vi "Frame Configuration Page.vi"(8 "error in (no error)":errorcluster, 11 "Node Ptr":T2 format="%.0x") -> (0 "error out":errorcluster)   [LabVIEW 2016, in "LIN Frame Protection Addon System Explorer.lvlib"]
uses:
  LIN Frame Protection Addon System Explorer.lvlib
  <vilib>/NI Veristand/Custom Device API/Custom Device Item Ref.ctl
  Shared/Types/Protection Type.ctl
  <vilib>/NI Veristand/Custom Device API/Custom Device API.lvlib
  Shared/LIN Frame Protection Addon Shared.lvlib
panel:
  in  "Protection Type":T1
  out "Frame ID":u32 format="%.0x"
  in  "Max Count":dbl=4.0
  out "Frame Rate":dbl
  out "Rolling Counter Channel":string
  out "CRC Channel":string
  in  "SHDocVw.IWebBrowser":refnum<k7>(container)
  in  "Value":dbl
  in  "Monitored Channels":i32(listbox)
  in  "Header":cluster{"Section Name":string}={"Section Name"="Custom Device Item Settings"}
  in  "Description":string
  in  "Name":string
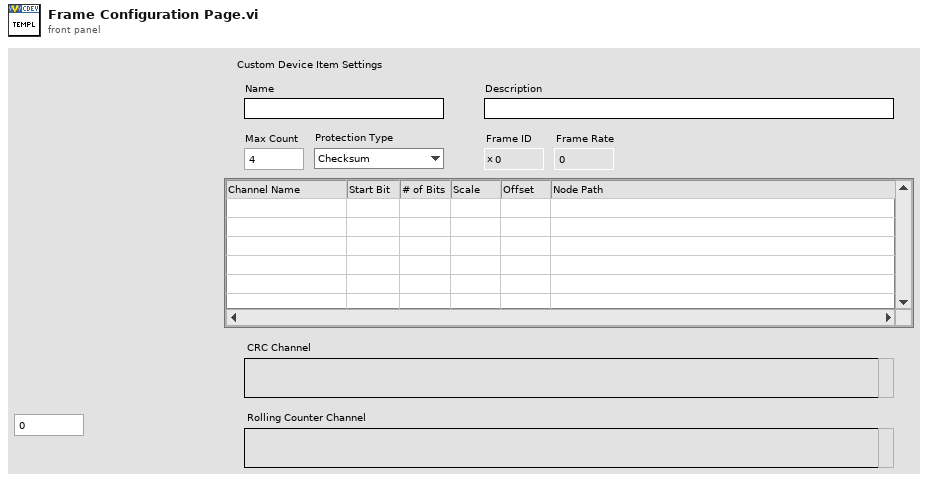
[diagram p1: front panel]
types:
  T1 = typedef "LIN Frame Protection Addon Shared.lvlib/Protection Type.ctl" = enum16{"Checksum", "CRC", "None (Counter Only)"}
  T2 = typedef "Custom Device API.lvlib/Custom Device Item Ref.ctl" = u64
  T3 = typedef "Custom Device API.lvlib/Custom Device Item Info.ctl" = cluster{"Name":string, "Is Channel":bool, "GUID":string, "Is Waveform":bool}
  T4 = typedef "LIN Frame Protection Addon Shared.lvlib/FrameConfiguration.ctl" = cluster{"Input Channels":T5[], "Schedule_SumOfDelays":dbl, "Rolling Counter Count":dbl, "PCL Count":u64, "Max Count":dbl, "Frame ID":u32, "Rolling Counter":T5, "CRC":T5, "Frame Name":string, "Cluster":string, "Database":string, "Protection Type":T1}
  T5 = typedef "LIN Frame Protection Addon Shared.lvlib/InputChannelConfiguration.ctl" = cluster{"Start Bit":i32, "Name":string, "Node Path":string, "Number of bits":i32, "Scale":dbl, "Offset":dbl, "Data Type":u32}
  T6 = typedef "Custom Device API.lvlib/Custom Device Commands.ctl" = enum16{"Default", "Item renamed", "Shutdown", "Dynamic button pressed"}
  T7 = typedef "LVPoint32TypeDef.ctl" = cluster{"Horizontal":i32, "Vertical":i32}
  T8 = typedef "LVRowAndColumnTypeDef.ctl" = cluster{"Row":i32, "Column":i32}
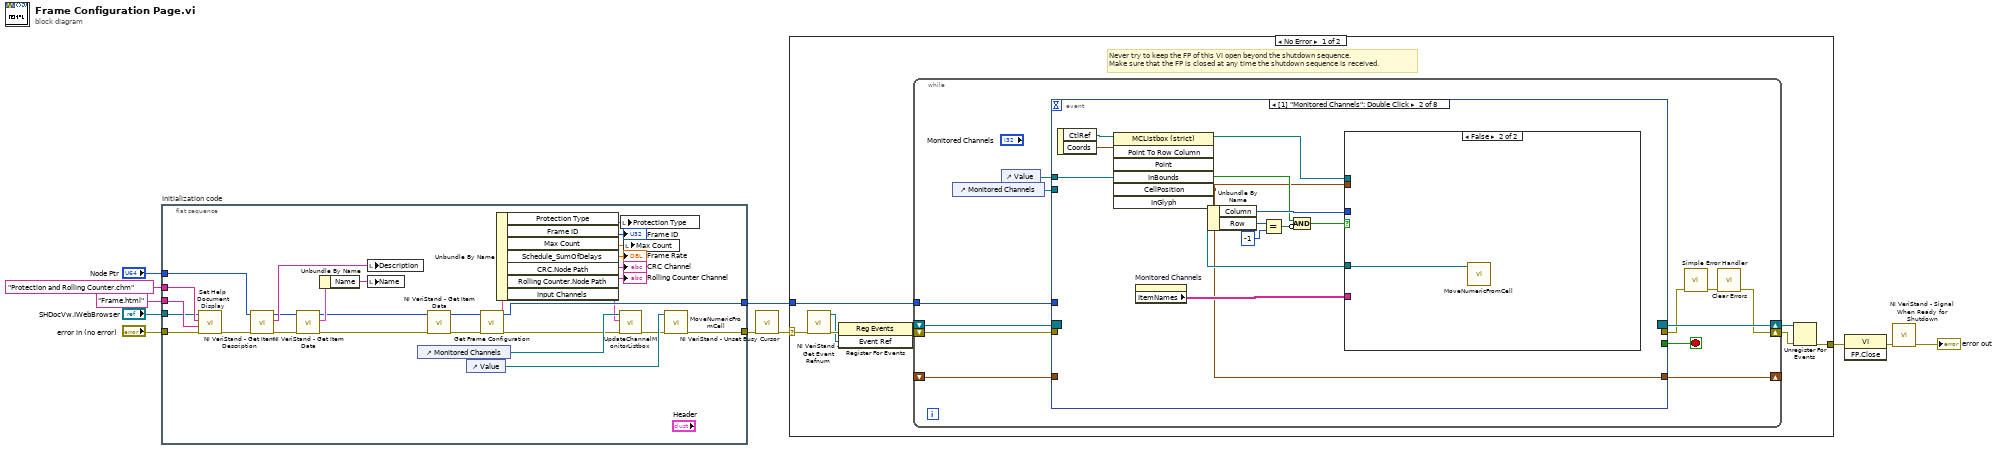
[diagram p0: block diagram]
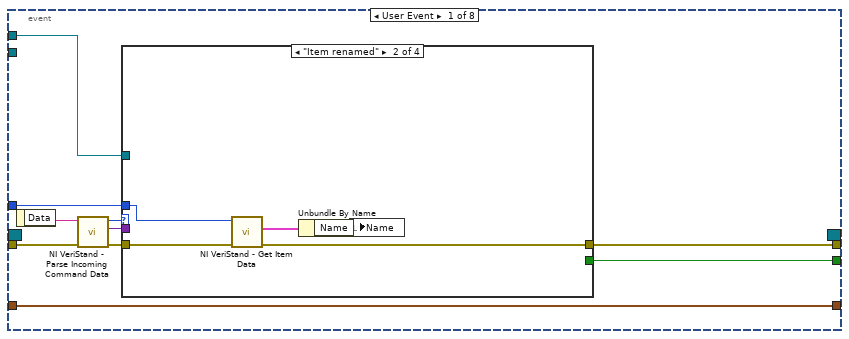
[diagram p2: hidden frame]
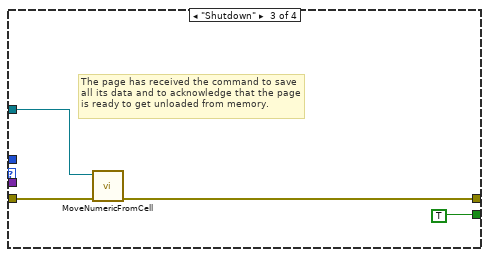
[diagram p4: hidden frame]
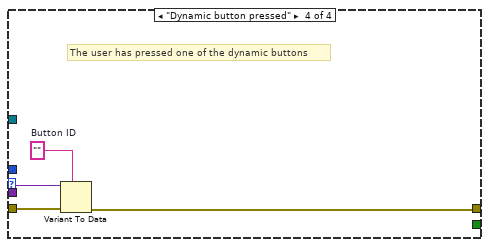
[diagram p5: hidden frame]
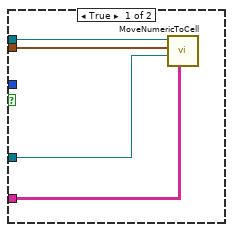
[diagram p6: hidden frame]
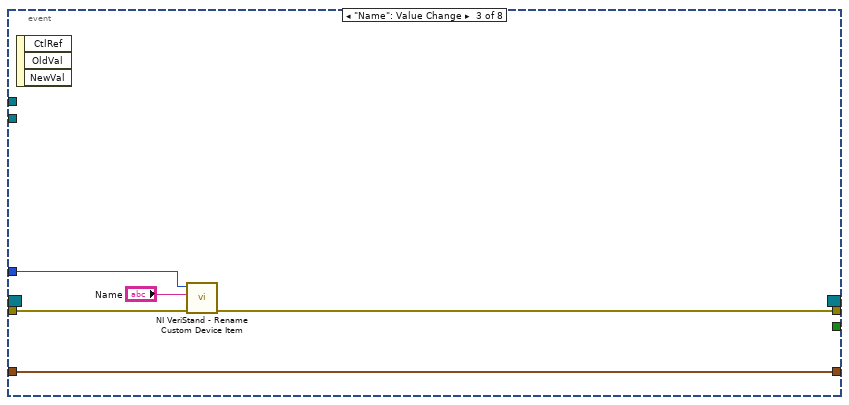
[diagram p7: hidden frame]
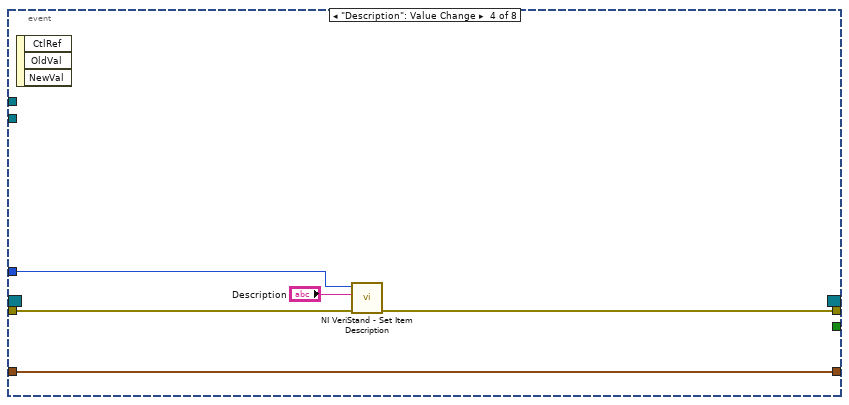
[diagram p8: hidden frame]
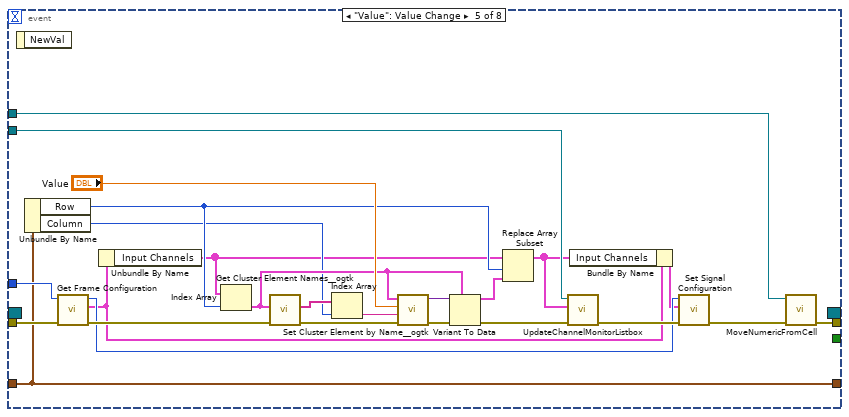
[diagram p9: hidden frame]
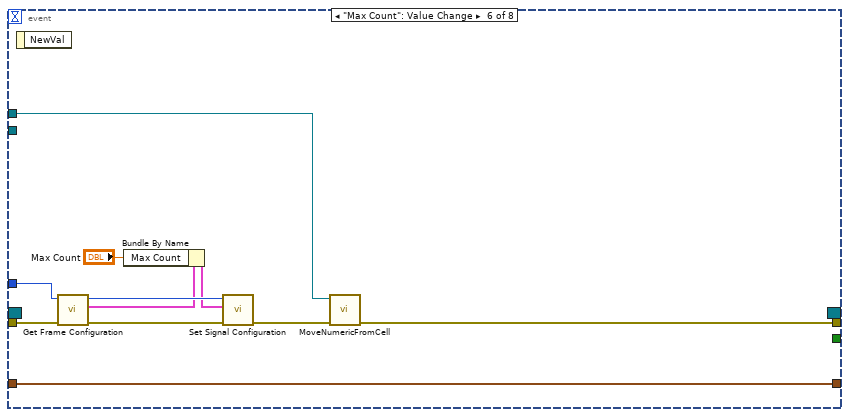
[diagram p10: hidden frame]
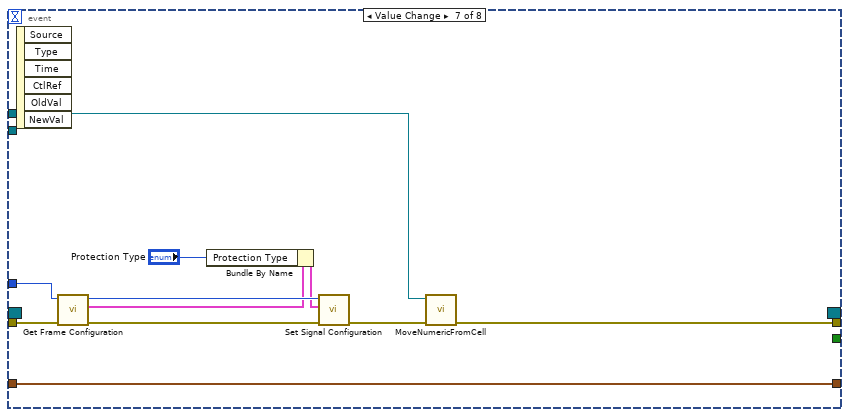
[diagram p11: hidden frame]
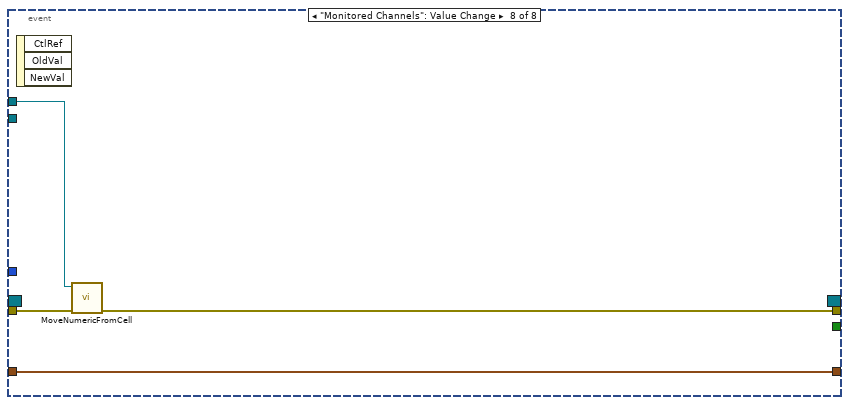
[diagram p12: hidden frame]
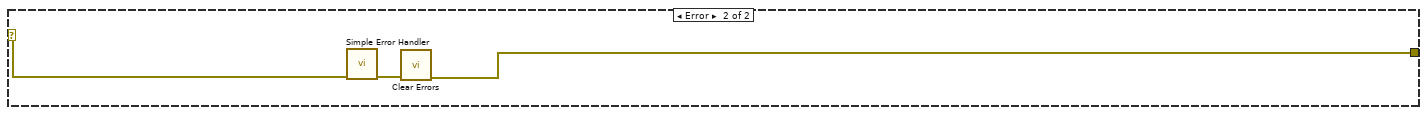
[diagram p13: hidden frame]
diagram:
  n1 = flat-sequence "Initialization code" {
    tunnel: "error in (no error)" -> [w31]
    tunnel: "Node Ptr" -> [w19]
    tunnel: [w28] -> w9
    tunnel: [w36] -> w7
    tunnel: "Protection and Rolling Counter.chm" ("Main CHM File") -> [w40]
    tunnel: "Frame.html" ("HTML File") -> [w39]
    tunnel: "SHDocVw.IWebBrowser" -> [w38]
    frame #0 {
      n2 = call "Set Help Document Display.vi"("error in (no error)"=w31, "HTML File"=w39, "Main CHM File"=w40, "SHDocVw.IWebBrowser2"=w38) -> ("error out"=w21:errorcluster)  [unwired: 7 in]
      n3 = call <vilib>:"NI VeriStand - Get Item Description.vi"("error in (no error)"=w21, "Item Ref in"=w19) -> ("error out"=w24:errorcluster, "Description"=w23:string, "Item Ref out"=w22:T2)  [unwired: 7 out]
      n4 = call <vilib>:"NI VeriStand - Get Item Data.vi"("error in (no error)"=w24, "Item Ref in"=w22) -> ("error out"=w20:errorcluster, "Item Info"=w25:T3, "Item Ref out"=w18:T2)  [unwired: 7 out]
      n5 = Unbundle By Name(w25) -> ("Name"=w26:string)
      n6 = local write "Description"(w23) -> ()
      n7 = local write "Name"(w26) -> ()
      n8 = control-ref of="Monitored Channels"() -> (w33:refnum<vi>)
      n9 = call <vilib>:"NI VeriStand - Get Item Data.vi"("error in (no error)"=w20, "Item Ref in"=w18) -> ("error out"=w35:errorcluster, "Item Ref out"=w37:T2)  [unwired: 8 out]
      n10 = control-ref of="Value"() -> (w30:refnum<vi>)
      n11 = call "Get Frame Configuration.vi"("error in"=w35, "Parent Ref"=w37) -> ("error out"=w32:errorcluster, "Selected Channels"=w34:T4, "Parent Ref Out"=w36:T2)  [unwired: 7 in]
      n12 = Unbundle By Name(w34) -> ("Protection Type"=w12:T1, "Frame ID"=→"Frame ID":u32, "Max Count"=w14:dbl, "Schedule_SumOfDelays"=→"Frame Rate":dbl, "CRC.Node Path"=→"CRC Channel":string, "Rolling Counter.Node Path"=→"Rolling Counter Channel":string, "Input Channels"=w27:T5[])
      n13 = call "UpdateChannelMonitorListbox.vi"("error in (no error)"=w32, "Monitored Channels"=w27, "Listbox"=w33) -> ("error out"=w29:errorcluster)  [unwired: 8 in]
      n14 = local write "Protection Type"(w12) -> ()
      n15 = local write "Max Count"(w14) -> ()
      n16 = call "MoveNumericFromCell.vi"("error in (no error)"=w29, "Digital in"=w30) -> ("error out"=w28:errorcluster)  [unwired: 9 in]
    }
  }
  n17 = call <vilib>:"NI VeriStand - Unset Busy Cursor.vi"("error in (no error)"=w9) -> ("error out"=w8:errorcluster)  [unwired: 10 out]
  n18 = case shown="No Error" w8 {
    selector: w8 -> [w41 w166]
    tunnel: [w46 w164] -> w11
    tunnel: w7 -> [w42 _]
    frame No Error {
      # "Never try to keep the FP of this VI open beyond the shutdown sequence.\nMake sure that the FP is closed at any time the shutdown sequence is received."
      n19 = call <vilib>:"NI VeriStand - Get Event Refnum.vi"("error in (no error)"=w41) -> ("error out"=w49:errorcluster, "Event Ref"=w45:refnum<user-event>)  [unwired: 9 out]
      n20 = register-events(error in=w49, w45) -> (reference out=w43:refnum<event-registration>, error out=w44:errorcluster)  [unwired: 1 in]
      n21 = while {
        tunnel: w42 -> [w57]
        shift-right: [w54] -> w47
        shift-left: w44 -> [w60]
        shift-right: [w61] -> w48
        shift-left: w43 -> [w59]
        shift-right: [w52] -> _
        shift-left: _ -> [w51]
        stop <- w58 stop-if-true
        n22 = control-ref of="Monitored Channels"() -> (w50:refnum<vi>)
        n23 = control-ref of="Value"() -> (w53:refnum<vi>)
        n24 = event shown="[1] \"Monitored Channels\": Double Click" {
          selector: w59 -> [_ _ _ _ _ _ _ _]
          dyn-events: [_ _ _ _ _ _ _ _] -> w61
          timeout: _ -> [_ _ _ _ _ _ _ _]
          tunnel: w60 -> [w71 _ w105 w110 w135 w146 w157 w161]
          tunnel: [w67 _ _ _ _ _ _ _] -> w58
          tunnel: [w66 _ w103 w109 w119 w143 w154 w160] -> w56
          tunnel: w57 -> [w65 _ w104 w108 w136 w147 w158 _]
          tunnel: w53 -> [w62 w93 _ _ w137 w148 w159 w162]
          tunnel: [w63 w86 w107 w112 w131 w144 w155 w163] -> w52
          tunnel: w51 -> [w63 _ w107 w112 w131 w144 w155 w163]
          tunnel: w50 -> [_ _ _ _ w134 _ _ _]
          event User Event {
            n25 = event-data() -> ("Data"=w70:string)  [unwired: 1 out]
            n26 = call <vilib>:"NI VeriStand - Parse Incoming Command Data.vi"("error in (no error)"=w71, "Incoming data"=w70) -> ("error out"=w69:errorcluster, "Outgoing data"=w64:variant, "Action"=w68:T6)  [unwired: 7 out]
            n27 = case shown="\"Item renamed\"" w68 {
              tunnel: w69 -> [w72 w75 w79 w85]
              tunnel: [_ _ TRUE _] -> w67
              tunnel: [w72 w74 w78 w82] -> w66
              tunnel: w65 -> [_ w73 _ _]
              tunnel: w64 -> [_ _ _ w84]
              tunnel: w62 -> [_ _ w80 _]
              frame "Default", Default {
              }
              frame "Item renamed" {
                n28 = call <vilib>:"NI VeriStand - Get Item Data.vi"("error in (no error)"=w75, "Item Ref in"=w73) -> ("error out"=w74:errorcluster, "Item Info"=w76:T3)  [unwired: 8 out]
                n29 = Unbundle By Name(w76) -> ("Name"=w77:string)
                n30 = local write "Name"(w77) -> ()
              }
              frame "Shutdown" {
                # "The page has received the command to save all its data and to acknowledge that the page is ready to get unloaded from memory."
                n31 = call "MoveNumericFromCell.vi"("error in (no error)"=w79, "Digital in"=w80) -> ("error out"=w78:errorcluster)  [unwired: 9 in]
              }
              frame "Dynamic button pressed" {
                w83 = ""  # Button ID
                # "The user has pressed one of the dynamic buttons"
                n32 = Variant To Data(error in=w85, type=w83, Variant=w84) -> (error out=w82:errorcluster)  [unwired: 1 out]
              }
            }
          }
          event "Monitored Channels": Double Click {
            n33 = event-data() -> ("CtlRef"=w96:refnum<vi>, "Coords"=w95:T7)  [unwired: 1 out]
            n34 = invoke class="MCListbox (strict)" method="Point To Row Column"(reference=w96, "Point"=w95) -> (reference out=w94:refnum<vi>, "InBounds"=w90:bool, "CellPosition"=w86:T8)  [unwired: 5 in, 4 out]
            n35 = property on="Monitored Channels" class="MCListbox (strict)"() -> ("ItemNames"=w87:string[][])  [unwired: 2 in, 2 out]
            n36 = Unbundle By Name(w86) -> ("Column"=w97:i32, "Row"=w91:i32)
            n37 = Equal?(x=w91, y=-1) -> (x = y?=w89:bool)
            n38 = Compound Arithmetic op=AND(w90, invert w89) -> (w88:bool)
            n39 = case shown="False" w88 {
              tunnel: w97 -> [_ _]
              tunnel: w94 -> [w101 _]
              tunnel: w86 -> [w100 _]
              tunnel: w93 -> [w99 w102]
              tunnel: w87 -> [w98 _]
              frame True {
                n40 = call "MoveNumericToCell.vi"("Data"=w98, "Numeric"=w99, "Cell Position"=w100, "Listbox"=w101) -> ()  [unwired: 7 in, 1 out]
              }
              frame False {
                n41 = call "MoveNumericFromCell.vi"("Digital in"=w102) -> ()  [unwired: 10 in, 1 out]
              }
            }
          }
          event "Name": Value Change {
            n42 = event-data() -> ()  [unwired: 4 out]
            n43 = call <vilib>:"NI VeriStand - Rename Custom Device Item.vi"("error in (no error)"=w105, "New Name"="Name", "Item Ref in"=w104) -> ("error out"=w103:errorcluster)  [unwired: 1 in, 7 out]
          }
          event "Description": Value Change {
            n44 = event-data() -> ()  [unwired: 4 out]
            n45 = call <vilib>:"NI VeriStand - Set Item Description.vi"("error in (no error)"=w110, "Description"="Description", "Item Ref in"=w108) -> ("error out"=w109:errorcluster)  [unwired: 8 out]
          }
          event "Value": Value Change {
            n46 = event-data() -> ()  [unwired: 2 out]
            n47 = Unbundle By Name(w131) -> ("Row"=w120:i32, "Column"=w118:i32)
            n48 = call "Get Frame Configuration.vi"("error in"=w135, "Parent Ref"=w136) -> ("error out"=w124:errorcluster, "Selected Channels"=w115:T4, "Parent Ref Out"=w117:T2)  [unwired: 7 in]
            n49 = Unbundle By Name(w115) -> ("Input Channels"=w116:T5[])
            n50 = Index Array(array=w116, index=w120) -> (element=w122:T5)
            n51 = call <userlib>:"Get Cluster Element Names__ogtk.vi"("error in (no error)"=w124, "Cluster"=w122) -> ("error out"=w125:errorcluster, "Element Names"=w130:string[])  [unwired: 8 in]
            n52 = Index Array(array=w130, index=w118) -> (element=w129:string)
            n53 = call <userlib>:"Set Cluster Element by Name__ogtk.vi"("error in (no error)"=w125, "Element Name (\"\": New Element Data Name)"=w129, "New Element Value"="Value", "Cluster"=w122) -> ("error out"=w126:errorcluster, "VCluster out"=w127:variant)  [unwired: 5 in, 1 out]
            n54 = Variant To Data(error in=w126, type=w122, Variant=w127) -> (data=w121:T5, error out=w123:errorcluster)
            n55 = Replace Array Subset(array=w116, new element=w121, index=w120) -> (w114:T5[])
            n56 = call "UpdateChannelMonitorListbox.vi"("error in (no error)"=w123, "Monitored Channels"=w114, "Listbox"=w134) -> ("error out"=w133:errorcluster)  [unwired: 8 in]
            n57 = Bundle By Name(cluster=w115, "Input Channels"=w114) -> (w113:T4)
            n58 = call "Set Signal Configuration.vi"("error in"=w133, "Selected Channels"=w113, "Parent Ref"=w117) -> ("error out"=w132:errorcluster)  [unwired: 7 in, 1 out]
            n59 = call "MoveNumericFromCell.vi"("error in (no error)"=w132, "Digital in"=w137) -> ("error out"=w119:errorcluster)  [unwired: 9 in]
          }
          event "Max Count": Value Change {
            n60 = event-data() -> ()  [unwired: 2 out]
            n61 = call "Get Frame Configuration.vi"("error in"=w146, "Parent Ref"=w147) -> ("error out"=w139:errorcluster, "Selected Channels"=w141:T4, "Parent Ref Out"=w142:T2)  [unwired: 7 in]
            n62 = Bundle By Name(cluster=w141, "Max Count"="Max Count") -> (w140:T4)
            n63 = call "Set Signal Configuration.vi"("error in"=w139, "Selected Channels"=w140, "Parent Ref"=w142) -> ("error out"=w145:errorcluster)  [unwired: 7 in, 1 out]
            n64 = call "MoveNumericFromCell.vi"("error in (no error)"=w145, "Digital in"=w148) -> ("error out"=w143:errorcluster)  [unwired: 9 in]
          }
          event Value Change {
            n65 = event-data() -> ()  [unwired: 7 out]
            n66 = call "Get Frame Configuration.vi"("error in"=w157, "Parent Ref"=w158) -> ("error out"=w150:errorcluster, "Selected Channels"=w152:T4, "Parent Ref Out"=w153:T2)  [unwired: 7 in]
            n67 = Bundle By Name(cluster=w152, "Protection Type"="Protection Type") -> (w151:T4)
            n68 = call "Set Signal Configuration.vi"("error in"=w150, "Selected Channels"=w151, "Parent Ref"=w153) -> ("error out"=w156:errorcluster)  [unwired: 7 in, 1 out]
            n69 = call "MoveNumericFromCell.vi"("error in (no error)"=w156, "Digital in"=w159) -> ("error out"=w154:errorcluster)  [unwired: 9 in]
          }
          event "Monitored Channels": Value Change {
            n70 = event-data() -> ()  [unwired: 4 out]
            n71 = call "MoveNumericFromCell.vi"("error in (no error)"=w161, "Digital in"=w162) -> ("error out"=w160:errorcluster)  [unwired: 9 in]
          }
        }
        n72 = call <vilib>:"Simple Error Handler.vi"("error in (no error)"=w56) -> ("error out"=w55:errorcluster)  [unwired: 1 in, 7 out]
        n73 = call <vilib>:"Clear Errors.vi"("error in (no error)"=w55) -> ("error out"=w54:errorcluster)  [unwired: 1 in, 5 out]
      }
      n74 = Unregister For Events(event registration refnum=w48, error in=w47) -> (error out=w46:errorcluster)
    }
    frame Error {
      n75 = call <vilib>:"Simple Error Handler.vi"("error in (no error)"=w166) -> ("error out"=w165:errorcluster)  [unwired: 1 in, 7 out]
      n76 = call <vilib>:"Clear Errors.vi"("error in (no error)"=w165) -> ("error out"=w164:errorcluster)  [unwired: 1 in, 5 out]
    }
  }
  n77 = invoke class="VI" method="FP.Close"(error in=w11) -> (error out=w10:errorcluster)  [unwired: 2 in, 2 out]
  n78 = call <vilib>:"NI VeriStand - Signal When Ready for Shutdown.vi"("error in (no error)"=w10) -> ("error out"=→"error out":errorcluster)  [unwired: 10 out]
